vi "Main.vi"(8 "error in (no error)":errorcluster, 11 "Waveform in":refnum<class "Waveform.lvclass">) -> (0 "error out":errorcluster, 3 "component":refnum<class "Waveform.lvclass">)   [LabVIEW 2012, in "Waveform.lvclass"]
doc: "Main VI of the component. This should contain the GUI of your component and be called when creating an executable."
uses:
  Waveform.lvclass
  PC_wavelength.ctl
  Waveform.lvclass/Waveform.ctl
  <vilib>/Distrio/Murmex/InitialiseMessage/InitialiseMessage.lvclass
  <vilib>/Distrio/Murmex/Murmex/update_cluster.ctl
  <vilib>/Distrio/Murmex/ConfigureMessage/ConfigureMessage.lvclass
  <vilib>/Distrio/Murmex/StopMessage/StopMessage.lvclass
  <vilib>/Distrio/Murmex/StartMessage/StartMessage.lvclass
  <vilib>/Distrio/Murmex/StartMessage/run mode enum.ctl
  <vilib>/Distrio/Murmex/TerminateMessage/TerminateMessage.lvclass
  <vilib>/Distrio/Murmex/Murmex/Set configure at initialise.vi
  <vilib>/Distrio/Murmex/Murmex/Set VI reference.vi
  <vilib>/Distrio/Murmex/Murmex/Get ID.vi
  <vilib>/Distrio/Murmex/Murmex/Set relay start stop to observers.vi
  <vilib>/Distrio/Murmex/Murmex/Set log reference.vi
  <vilib>/Distrio/Murmex/Murmex/Set license required.vi
  <vilib>/Distrio/Murmex/Murmex/Set write log to disk.vi
  <vilib>/Distrio/Murmex/StartMessage/Set run mode.vi
  <vilib>/Distrio/Murmex/Murmex/Murmex.lvclass
panel:
  out "terminate?":bool=TRUE
  in  "button::quit":bool
  in  "button:start_finite":bool
  in  "button:start_free-run":bool
  in  "button::configure":bool
  in  "Tab Control":enum32{"Waveforms", "Debug", "Graphs"}(tab)
  in  "Illumination arm":enum16{"Florence", "Prato"}(ring)
  in  "Delay 2":dbl[unit] caption="delay" step=1e-06
  in  "Offset 2":dbl[unit] caption="offset" min=-5.0 max=5.0 step=0.01
  in  "Amplitude 2":dbl[unit]=1.0 caption="amplitude" min=0.0 max=5.0 step=0.01
  in  "Delay 1":dbl[unit] caption="delay" step=1e-06
  in  "Offset 1":dbl[unit] caption="offset" min=-5.0 max=5.0 step=0.01
  in  "Amplitude 1":dbl[unit]=1.0 caption="amplitude" min=0.0 max=5.0 step=0.01
  in  "Wavelength":T1 items=["405nm"=0.48, "445nm"=0.52, "491nm"=0.58, "515nm"=0.6, "561nm"=0.66]
  out "Counter2":dbl[unit]
  out "Counter1":dbl[unit]
  in  "ID":string="waveform"
  out "HSYNC pulses":i32=2048 min=4 max=2048 step=4
  out "frame rate":dbl[unit]=100.0
  out "Mixed Signal Graph":T2(graph)
  out "log":string
  # "Pockels Cell"
  # "galvo 1"
  # "galvo 2"
  # "Orca"
  # "actual frequencies"
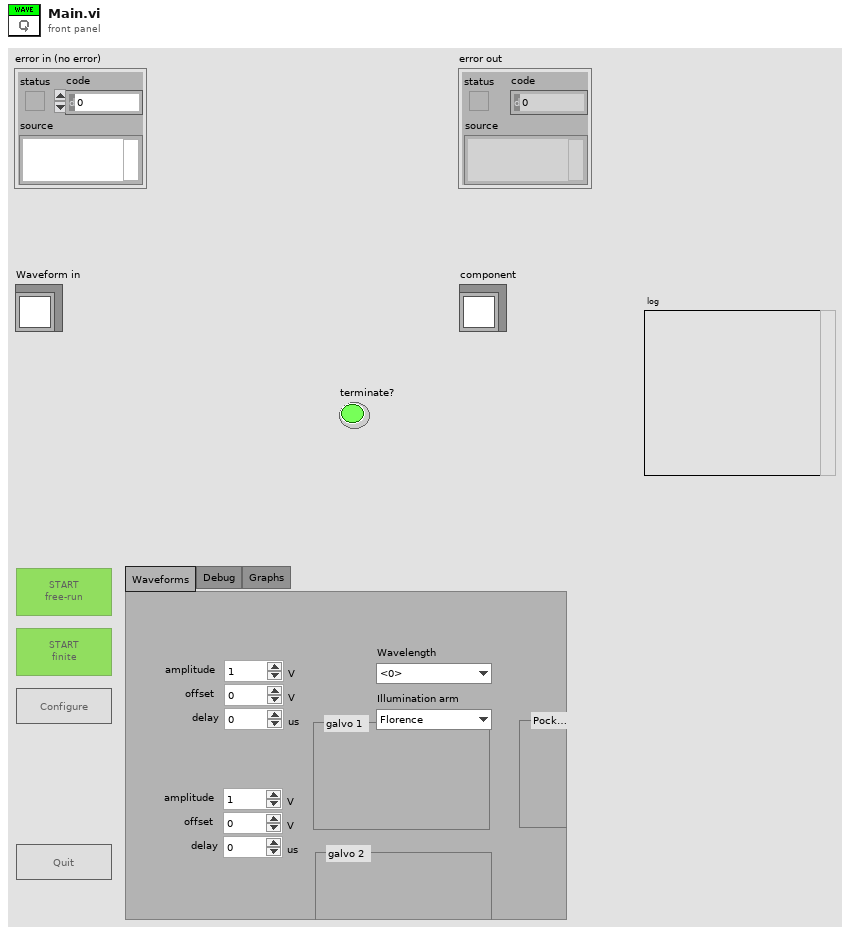
[diagram p1: front panel]
types:
  T1 = typedef "PC_wavelength.ctl" = dbl
  T2 = cluster{"galvo1 waveform":waveform(dbl), "galvo2 waveform":waveform(dbl), dbl[]}
  T3 = typedef "Murmex.lvlib/Murmex.lvclass/update_cluster.ctl" = cluster{"target ID":string, "key chains":string[], "values":variant[]}
  T4 = typedef "Murmex.lvlib/StartMessage.lvclass/run mode enum.ctl" = enum16{"infinite", "finite"}
  T5 = enum8{"Enabled", "Disabled", "Disabled and Grayed Out"}
  T6 = typedef "Murmex.lvlib/Murmex.lvclass/command_enum.ctl" = enum16{"null", "initialise", "reset", "terminate", "acknowledge", "update", "inspect", "inform", "proceed", "start", "stop", "fetch", "configure", "generic"}
  T7 = typedef "Murmex.lvlib/Murmex.lvclass/Event type enumerations.ctl" = enum16{"before", "after"}
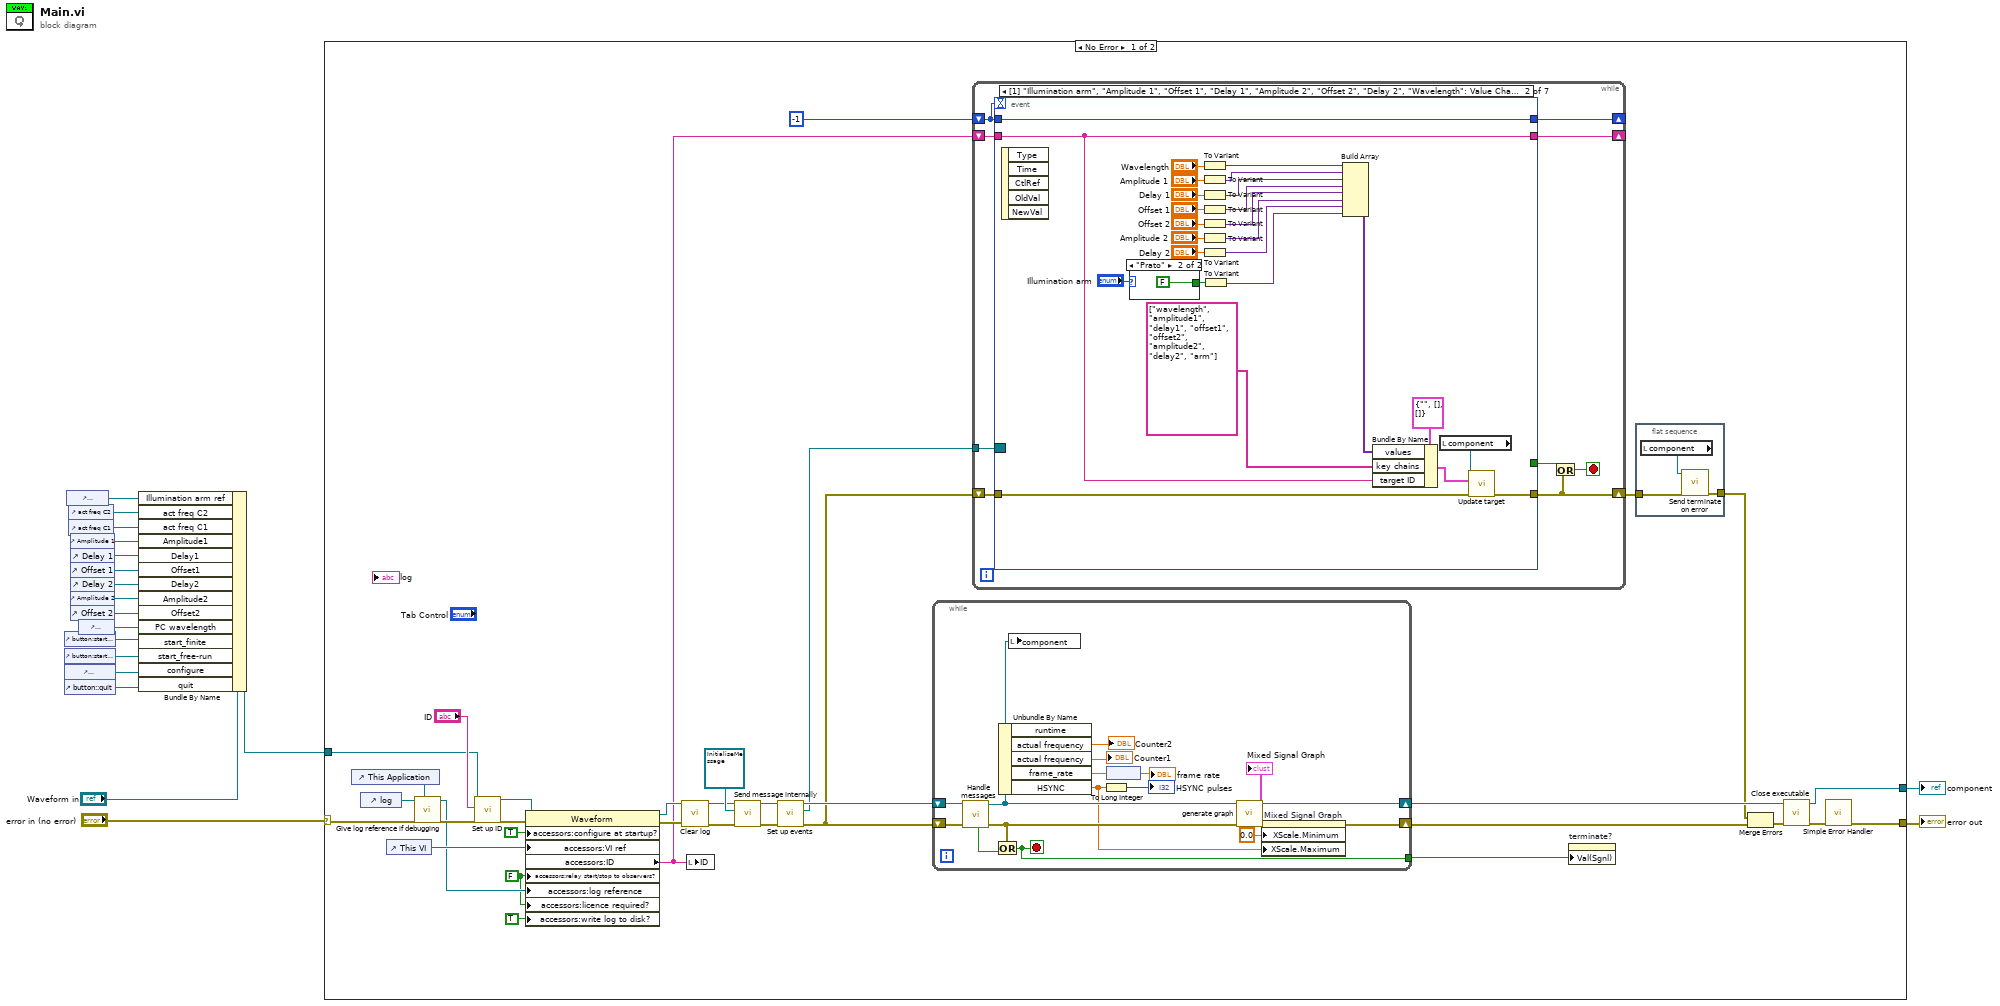
[diagram p0: block diagram]
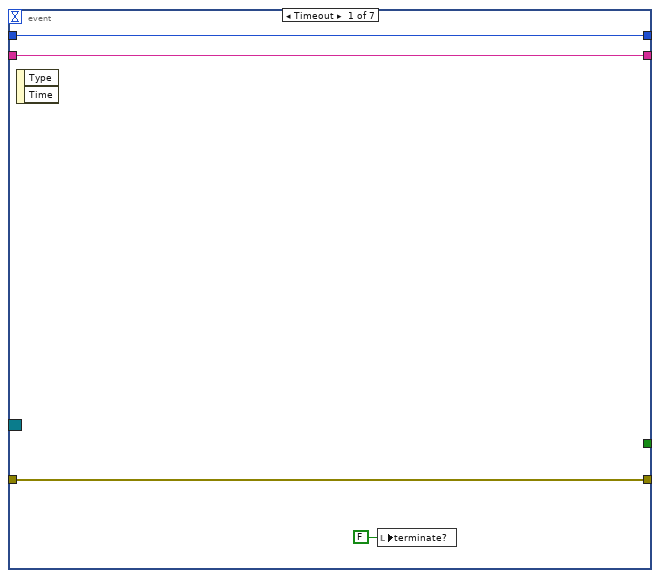
[diagram p2: hidden frame]
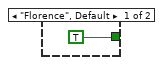
[diagram p3: hidden frame]
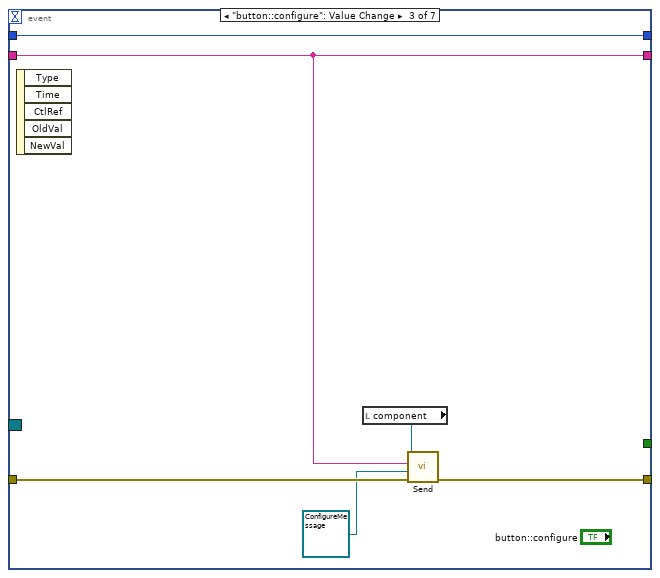
[diagram p4: hidden frame]
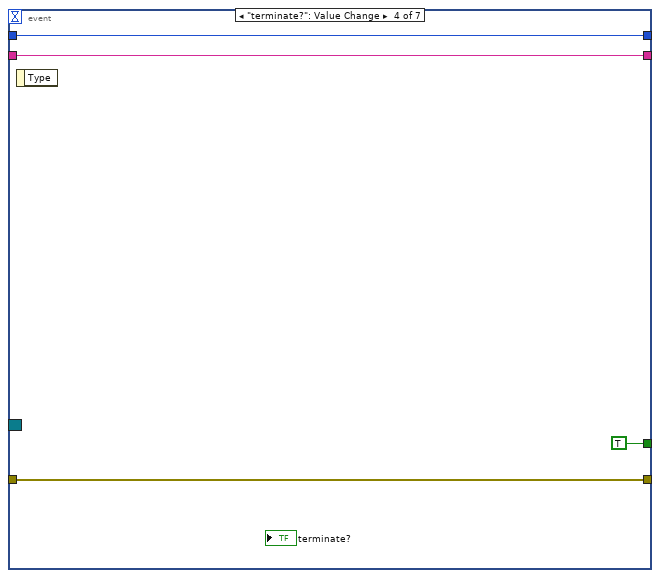
[diagram p5: hidden frame]
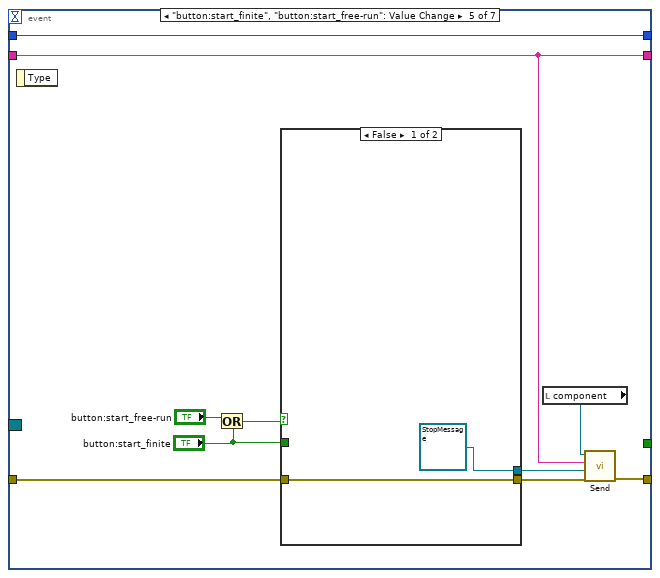
[diagram p6: hidden frame]
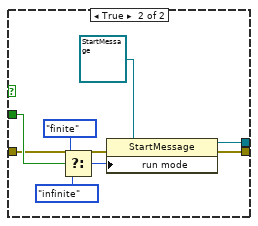
[diagram p7: hidden frame]
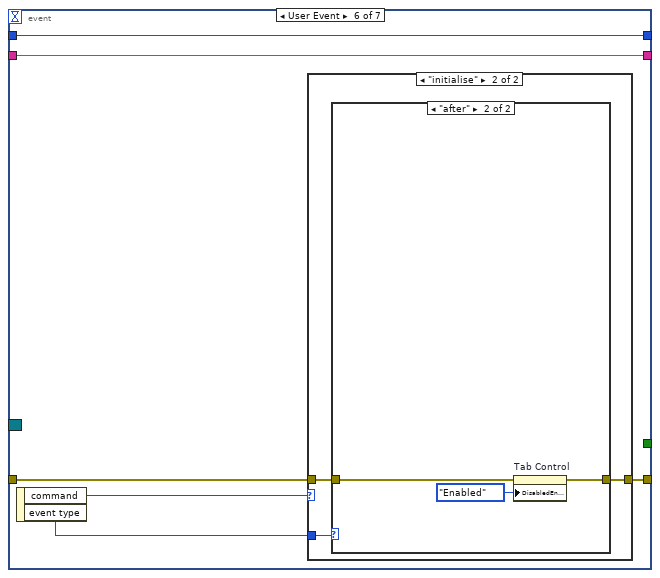
[diagram p8: hidden frame]
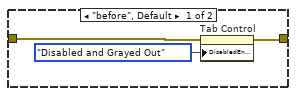
[diagram p10: hidden frame]
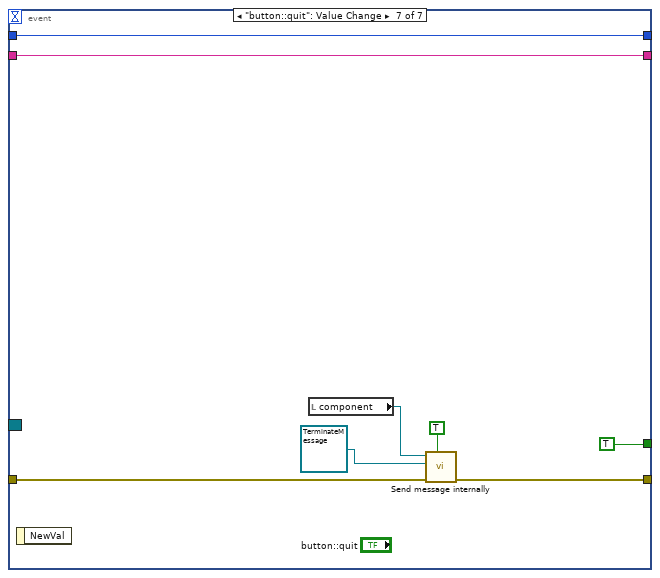
[diagram p11: hidden frame]
diagram:
  n1 = control-ref of="button:start_finite"() -> (w11:refnum<vi>)
  n2 = control-ref of="button:start_free-run"() -> (w12:refnum<vi>)
  n3 = control-ref of="button::configure"() -> (w13:refnum<vi>)
  n4 = control-ref of="button::quit"() -> (w14:refnum<vi>)
  n5 = control-ref of="Illumination arm"() -> (w1:refnum<vi>)
  n6 = control-ref of="act freq C2"() -> (w2:refnum<vi>)
  n7 = control-ref of="act freq C1"() -> (w3:refnum<vi>)
  n8 = control-ref of="Amplitude 1"() -> (w4:refnum<vi>)
  n9 = control-ref of="Delay 1"() -> (w5:refnum<vi>)
  n10 = control-ref of="Offset 1"() -> (w6:refnum<vi>)
  n11 = control-ref of="Delay 2"() -> (w7:refnum<vi>)
  n12 = control-ref of="Amplitude 2"() -> (w8:refnum<vi>)
  n13 = control-ref of="Offset 2"() -> (w9:refnum<vi>)
  n14 = control-ref of="Wavelength"() -> (w10:refnum<vi>)
  n15 = Bundle By Name(cluster="Waveform in", "Illumination arm ref"=w1, "act freq C2"=w2, "act freq C1"=w3, "Amplitude1"=w4, "Delay1"=w5, "Offset1"=w6, "Delay2"=w7, "Amplitude2"=w8, "Offset2"=w9, "PC wavelength"=w10, "start_finite"=w11, "start_free-run"=w12, "configure"=w13, "quit"=w14) -> (w17:refnum<class "Waveform.lvclass">)
  n16 = case shown="No Error" "error in (no error)" {
    selector: "error in (no error)" -> [w51 w170]
    tunnel: w17 -> [w48 w169]
    tunnel: [w29 w170] -> w16
    tunnel: [w28 w169] -> w15
    frame No Error {
      w42 = FALSE ("relay start/stop to observers?")
      n17 = control-ref of="This Application"() -> (w53:refnum<vi>)
      n18 = control-ref of="log"() -> (w52:refnum<vi>)
      n19 = control-ref of="This VI"() -> (w44:refnum<vi>)
      n20 = call "Give log reference if debugging.vi"("application ref"=w53, "error in (no error)"=w51, "log reference in"=w52) -> ("error out"=w50:errorcluster, "log reference out"=w43:refnum<vi>)  [unwired: 6 in, 1 out]
      n21 = call <vilib>:"Set up ID.vi"("error in (no error)"=w50, "component ID"="ID", "MurmexBase in"=w48) -> ("error out"=w47:errorcluster, "MurmexBase out"=w46:refnum<class "Waveform.lvclass">)  [unwired: 6 in, 1 out]
      n22 = property class="Waveform"(reference=w46, error in=w47, "accessors:configure at startup?"=TRUE ("configure at startup?"), "accessors:VI ref"=w44, "accessors:relay start/stop to observers?"=w42, "accessors:log reference"=w43, "accessors:licence required?"=w42, "accessors:write log to disk?"=TRUE ("write log to disk?")) -> (reference out=w34:refnum<class "Waveform.lvclass">, error out=w35:errorcluster, "accessors:ID"=w23:string)
      n23 = call <vilib>:"Clear log.vi"("error in (no error)"=w35, "MurmexBase in"=w34) -> ("error out"=w36:errorcluster, "MurmexBase out"=w37:refnum<class "Waveform.lvclass">)  [unwired: 8 in]
      n24 = local write "ID"(w23) -> ()
      n25 = call <vilib>:"Send message internally.vi"("error in (no error)"=w36, "Message"=refnum<class "InitialiseMessage.lvclass"> refnum ("Murmex.lvlib:InitialiseMessage"), "Murmex in"=w37) -> ("error out"=w39:errorcluster, "Murmex out"=w40:refnum<class "Waveform.lvclass">)  [unwired: 7 in]
      n26 = call <vilib>:"Set up events.vi"("error in (no error)"=w39, "MurmexBase in"=w40) -> ("error out"=w25:errorcluster, "Event Registration Refnum"=w24:refnum<event-registration>, "MurmexBase out"=w33:refnum<class "Waveform.lvclass">)  [unwired: 7 in]
      n27 = while {
        shift-right: [w155] -> w30
        shift-left: w25 -> [w168]
        shift-right: [w160] -> w27
        shift-left: w33 -> [w167]
        tunnel: [w163] -> w20
        stop <- w163 stop-if-true
        n28 = call <vilib>:"Handle messages.vi"("error in (no error)"=w168, "Murmex in"=w167) -> ("error out"=w162:errorcluster, "Murmex out"=w161:refnum<class "Waveform.lvclass">, "terminated?"=w166:bool)  [unwired: 7 in]
        n29 = Or(x=w162, y=w166) -> (x .or. y?=w163:bool)
        n30 = Unbundle By Name(w161) -> ("actual frequency"=→"Counter2":dbl[unit], "actual frequency"=→"Counter1":dbl[unit], "frame_rate"=w165:dbl, "HSYNC"=w153:dbl)  [unwired: 1 out]
        n31 = local write "component"(w161) -> ()
        n32 = To Long Integer(number=w153) -> (32bit integer=→"HSYNC pulses":i32)
        n33 = node(w165) -> (→"frame rate":dbl[unit])
        n34 = call-dynamic "generate graph.vi"("error in (no error)"=w162, "Waveform in"=w161) -> ("error out"=w156:errorcluster, "Mixed Signal Graph"=→"Mixed Signal Graph":T2, "Waveform out"=w160:refnum<class "Waveform.lvclass">)  [unwired: 7 in]
        n35 = property on="Mixed Signal Graph" class="MixedGraph (strict)"(error in=w156, "XScale.Minimum"=0.0 ("X Scale.Range:Minimum"), "XScale.Maximum"=w153) -> (error out=w155:errorcluster)  [unwired: 1 in, 1 out]
      }
      n36 = while {
        shift-right: [w63] -> _
        shift-left: -1 -> [w65]
        shift-right: [w61] -> w22
        shift-left: w25 -> [w62]
        tunnel: w24 -> [w64]
        shift-right: [w57] -> _
        shift-left: w23 -> [w58]
        stop <- w60 stop-if-true
        n37 = event shown="[1] \"Illumination arm\", \"Amplitude 1\", \"Offset 1\", \"Delay 1\", \"Amplitude 2\", \"Offset 2\", \"Delay 2\", \"Wavelength\": Value Change" {
          selector: w64 -> [_ _ _ _ _ _ _]
          dyn-events: _ -> [_ _ _ _ _ _ _]
          timeout: w65 -> [_ _ _ _ _ _ _]
          tunnel: w65 -> [w68 w90 w99 w107 w117 w133 w145]
          tunnel: [w68 w90 w99 w107 w117 w133 w145] -> w63
          tunnel: w62 -> [w69 w92 w103 w106 w113 w131 w150]
          tunnel: [w69 w95 w102 w106 w116 w128 w149] -> w61
          tunnel: [_ _ _ TRUE ("configure at startup?") _ _ TRUE] -> w59
          tunnel: [w67 w91 w98 w104 w114 w132 w144] -> w57
          tunnel: w58 -> [w67 w91 w98 w104 w114 w132 w144]
          event Timeout {
            n38 = event-data() -> ()  [unwired: 1 in, 2 out]
            n39 = local write "terminate?"(FALSE ("terminate?")) -> ()
          }
          event "Illumination arm", "Amplitude 1", "Offset 1", "Delay 1", "Amplitude 2", "Offset 2", "Delay 2": Value Change {
            n40 = event-data() -> ()  [unwired: 1 in, 5 out]
            n41 = case shown="\"Prato\"" "Illumination arm" {
              tunnel: [TRUE FALSE] -> w71
              frame "Florence", Default {
              }
              frame "Prato" {
              }
            }
            n42 = To Variant(anything="Wavelength") -> (Variant=w88:variant)
            n43 = To Variant(anything="Amplitude 1") -> (Variant=w78:variant)
            n44 = To Variant(anything="Delay 1") -> (Variant=w77:variant)
            n45 = To Variant(anything="Offset 1") -> (Variant=w76:variant)
            n46 = To Variant(anything="Offset 2") -> (Variant=w75:variant)
            n47 = To Variant(anything="Amplitude 2") -> (Variant=w74:variant)
            n48 = To Variant(anything="Delay 2") -> (Variant=w73:variant)
            n49 = To Variant(anything=w71) -> (Variant=w70:variant)
            n50 = Build Array(w88, w78, w77, w76, w75, w74, w73, w70) -> (w87:variant[])
            n51 = Bundle By Name(cluster=T3 {"target ID"="", "key chains"=[], "values"=[]} ("update cluster"), "values"=w87, "key chains"=string[] ["wavelength", "amplitude1", "delay1", "offset1", "offset2", "amplitude2", "delay2", "arm"], "target ID"=w91) -> (w93:T3)
            n52 = local read "component"() -> (w89:refnum<class "Waveform.lvclass">)
            n53 = call <vilib>:"Update target.vi"("error in (no error)"=w92, "update cluster"=w93, "MurmexBase in"=w89) -> ("error out"=w95:errorcluster)  [unwired: 7 in, 1 out]
          }
          event "button::configure": Value Change {
            n54 = event-data() -> ()  [unwired: 1 in, 5 out]
            n55 = local read "component"() -> (w101:refnum<class "Waveform.lvclass">)
            n56 = call <vilib>:"Send.vi"("error in (no error)"=w103, "Message"=refnum<class "ConfigureMessage.lvclass"> refnum ("Murmex.lvlib:ConfigureMessage"), "recipient"=w98, "Murmex in"=w101) -> ("error out"=w102:errorcluster)  [unwired: 6 in, 1 out]
          }
          event "terminate?": Value Change {
            n57 = event-data() -> ()  [unwired: 1 in, 1 out]
          }
          event "button:start_finite", "button:start_free-run": Value Change {
            n58 = event-data() -> ()  [unwired: 1 in, 1 out]
            n59 = Or(x="button:start_free-run", y="button:start_finite") -> (x .or. y?=w110:bool)
            n60 = case shown="False" w110 {
              tunnel: w113 -> [w119 w126]
              tunnel: [w119 w125] -> w112
              tunnel: [refnum<class "StopMessage.lvclass"> refnum ("Murmex.lvlib:StopMessage") w123] -> w111
              tunnel: "button:start_finite" -> [_ w127]
              frame False {
              }
              frame True {
                n61 = Select(t=run_mode_enum."finite" ("run mode"), s=w127, f=run_mode_enum."infinite" ("run mode")) -> (s? t:f=w122:T4)
                n62 = property class="StartMessage"(reference=refnum<class "StartMessage.lvclass"> refnum ("Murmex.lvlib:StartMessage"), error in=w126, "run mode"=w122) -> (reference out=w123:refnum<class "StartMessage.lvclass">, error out=w125:errorcluster)
              }
            }
            n63 = local read "component"() -> (w115:refnum<class "Waveform.lvclass">)
            n64 = call <vilib>:"Send.vi"("error in (no error)"=w112, "Message"=w111, "recipient"=w114, "Murmex in"=w115) -> ("error out"=w116:errorcluster)  [unwired: 6 in, 1 out]
          }
          event User Event {
            n65 = event-data() -> ("command"=w130:T6, "event type"=w129:T7)  [unwired: 1 in]
            n66 = case shown="\"initialise\"" w130 {
              tunnel: w131 -> [w134 w136]
              tunnel: w129 -> [_ w137]
              tunnel: [w134 w135] -> w128
              frame "null", Default {
              }
              frame "initialise" {
                n67 = case shown="\"after\"" w137 {
                  tunnel: w136 -> [w138 w143]
                  tunnel: [w139 w142] -> w135
                  frame "before", Default {
                    n68 = property on="Tab Control" class="TabCtl (strict)"(error in=w138, "DisabledEnum"=T5."Disabled and Grayed Out" ("Disabled")) -> (error out=w139:errorcluster)  [unwired: 1 in, 1 out]
                  }
                  frame "after" {
                    n69 = property on="Tab Control" class="TabCtl (strict)"(error in=w143, "DisabledEnum"=T5."Enabled" ("Disabled")) -> (error out=w142:errorcluster)  [unwired: 1 in, 1 out]
                  }
                }
              }
            }
          }
          event "button::quit": Value Change {
            n70 = event-data() -> ()  [unwired: 1 in, 1 out]
            n71 = local read "component"() -> (w148:refnum<class "Waveform.lvclass">)
            n72 = call <vilib>:"Send message internally.vi"("priority message? (F)"=TRUE, "error in (no error)"=w150, "Message"=refnum<class "TerminateMessage.lvclass"> refnum ("Murmex.lvlib:TerminateMessage"), "Murmex in"=w148) -> ("error out"=w149:errorcluster)  [unwired: 6 in, 1 out]
          }
        }
        n73 = Or(x=w59, y=w61) -> (x .or. y?=w60:bool)
      }
      n74 = property on="terminate?" class="Bool (strict)"("Val(Sgnl)"=w20) -> ()  [unwired: 2 in, 2 out]
      n75 = flat-sequence {
        tunnel: w22 -> [w56]
        tunnel: [w55] -> w21
        frame #0 {
          n76 = local read "component"() -> (w54:refnum<class "Waveform.lvclass">)
          n77 = call <vilib>:"Send terminate on error.vi"("error in (no error)"=w56, "Murmex in"=w54) -> ("error out"=w55:errorcluster)  [unwired: 8 in, 1 out]
        }
      }
      n78 = Merge Errors(w21, w30) -> (w31:errorcluster)
      n79 = call <vilib>:"Close executable.vi"("error in (no error)"=w31, "MurmexBase in"=w27) -> ("error out"=w32:errorcluster, "MurmexBase out"=w28:refnum<class "Waveform.lvclass">)  [unwired: 8 in]
      n80 = call <vilib>:"Simple Error Handler.vi"("error in (no error)"=w32) -> ("error out"=w29:errorcluster)  [unwired: 4 in, 4 out]
    }
    frame Error {
    }
  }
  "error out" <- w16
  "component" <- w15
